vi "Write Components.vi"(8 "error in (no error)":errorcluster, 10 "Components":T1[](array[typedef]), 11 "Snake in":refnum<class "Snake.lvclass">) -> (0 "error out":errorcluster, 3 "Snake out":refnum<class "Snake.lvclass">)   [LabVIEW 2019, in "Snake.lvclass"]
uses:
  Snake.lvclass
  Direction STYP.ctl
  Coordinate STYP.ctl
  private/Snake Component STYP.ctl
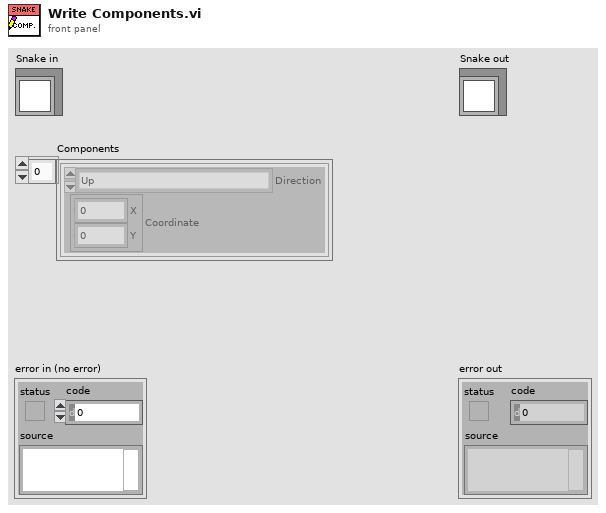
[diagram p1: front panel]
types:
  T1 = typedef "Snake.lvclass/Snake Component STYP.ctl" = cluster{"Direction":T2, "Coordinate":T3}
  T2 = typedef "Direction STYP.ctl" = enum16{"Up", "Down", "Left", "Right"}
  T3 = typedef "Coordinate STYP.ctl" = cluster{"X":i32, "Y":i32}
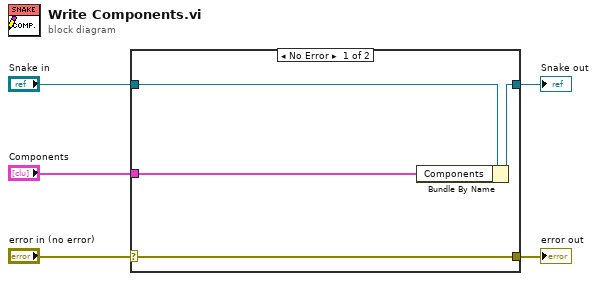
[diagram p0: block diagram]
diagram:
  n1 = case shown="No Error" "error in (no error)" {
    selector: "error in (no error)" -> [w9 w10]
    tunnel: [w9 w10] -> w4
    tunnel: [w7 w11] -> w2
    tunnel: "Snake in" -> [w8 w11]
    tunnel: "Components" -> [w6 _]
    frame No Error {
      n2 = Bundle By Name(cluster=w8, "Components"=w6) -> (w7:refnum<class "Snake.lvclass">)
    }
    frame Error {
    }
  }
  "error out" <- w4
  "Snake out" <- w2
